vi "normalize array.vi"(11 "u8_pxar_dist":u8[](array[numeric])) -> (3 "Array":dbl[](array[numeric]))   [LabVIEW 2011]
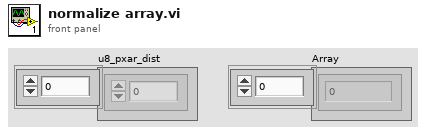
[diagram p1: front panel]
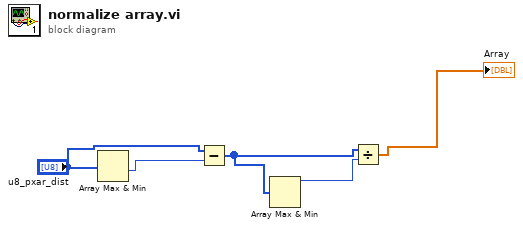
[diagram p0: block diagram]
diagram:
  n1 = Array Max & Min(array="u8_pxar_dist") -> (min value=w2:u8)  [unwired: 3 out]
  n2 = Subtract(x="u8_pxar_dist", y=w2) -> (x-y=w3:u8[])
  n3 = Array Max & Min(array=w3) -> (max value=w4:u8)  [unwired: 3 out]
  n4 = Divide(x=w3, y=w4) -> (x/y=→"Array":dbl[])
